vi "GetImageData.vi"(8 "error in (no error)":errorcluster, 11 "Image":T2) -> (0 "error out":errorcluster, 2 "ImageData Out":T1, 3 "Image out":T2)   [LabVIEW 2020]
uses:
  <vilib>/vision/Image Controls.llb/IMAQ Image.ctl
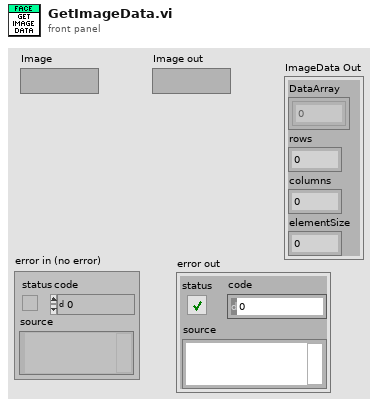
[diagram p1: front panel]
types:
  T1 = cluster{"DataArray":u8[], "rows":i32, "columns":i32, "elementSize":i32}
  T2 = typedef "IMAQ Image.ctl" = refnum<image>
  T3 = typedef "Image Type" = u32
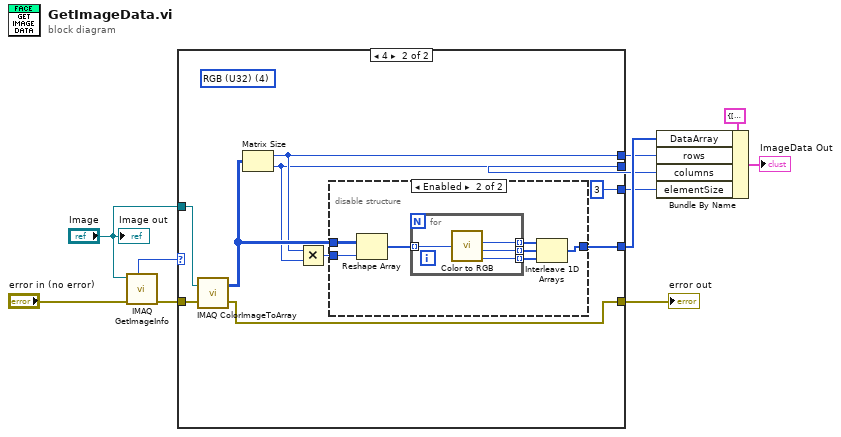
[diagram p0: block diagram]
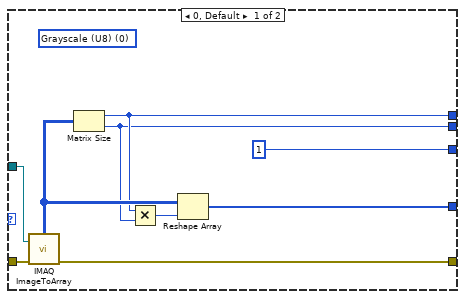
[diagram p2: hidden frame]
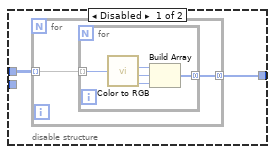
[diagram p3: hidden frame]
diagram:
  n1 = call "IMAQ GetImageInfo"("error in (no error)"="error in (no error)", "Image"="Image") -> ("error out"=w9:errorcluster, "Image Type"=w11:T3)  [unwired: 2 in, 6 out]
  n2 = case shown="4" w11 {
    tunnel: "Image" -> [w20 w29]
    tunnel: [w12 w28] -> w5
    tunnel: [1 3] -> w2
    tunnel: w9 -> [w18 w26]
    tunnel: [w17 w25] -> w7
    tunnel: [w14 w23] -> w4
    tunnel: [w13 w22] -> w3
    frame 0, Default {
      (unwired) T3 0 items=["Grayscale (U8)", "Grayscale (I16)", "Grayscale (SGL)", "Complex (CSG)", "RGB (U32)", "HSL (U32)", "RGB (U64)", "Grayscale (U16)"] ("Image Type")
      n3 = call "IMAQ ImageToArray"("error in (no error)"=w18, "Image"=w20) -> ("error out"=w17:errorcluster, "Image Pixels (U8)"=w16:u8[][])  [unwired: 2 in, 3 out]
      n4 = Matrix Size(0:w16) -> (1:w14:i32, 2:w13:i32)
      n5 = Multiply(x=w14, y=w13) -> (x*y=w15:i32)
      n6 = Reshape Array(w16, w15) -> (w12:u8[])
    }
    frame 4 {
      (unwired) T3 4 items=["Grayscale (U8)", "Grayscale (I16)", "Grayscale (SGL)", "Complex (CSG)", "RGB (U32)", "HSL (U32)", "RGB (U64)", "Grayscale (U16)"] ("Image Type")
      n7 = call "IMAQ ColorImageToArray"("Image"=w29, "error in (no error)"=w26) -> ("Image Pixels (U32)"=w24:u32[][], "error out"=w25:errorcluster)  [unwired: 2 in, 1 out]
      n8 = Matrix Size(0:w24) -> (1:w23:i32, 2:w22:i32)
      n9 = Multiply(x=w23, y=w22) -> (x*y=w21:i32)
      n10 = disable-structure shown="Enabled" {
        disable-tunnel: [w31 w39] -> w28
        disable-tunnel: w24 -> [w30 w45]
        disable-tunnel: w21 -> [_ w44]
        frame Disabled {
          n11 = for {
            tunnel: [w33] -> w31 mode=concatenating
            tunnel: w30 -> [w32] mode=indexing
            n12 = for {
              tunnel: w32 -> [w38] mode=indexing
              tunnel: [w34] -> w33 mode=concatenating
              n13 = call <vilib>:"Color to RGB.vi"("Color"=w38) -> ("R"=w37:u8, "G"=w36:u8, "B"=w35:u8)  [unwired: 1 out]
              n14 = Build Array(w37, w36, w35) -> (w34:u8[])
            }
          }
        }
        frame Enabled {
          n15 = Reshape Array(w45, w44) -> (w43:u32[])
          n16 = for {
            tunnel: w43 -> [w49] mode=indexing
            tunnel: [w48] -> w42 mode=indexing
            tunnel: [w47] -> w41 mode=indexing
            tunnel: [w46] -> w40 mode=indexing
            n17 = call <vilib>:"Color to RGB.vi"("Color"=w49) -> ("R"=w48:u8, "G"=w47:u8, "B"=w46:u8)  [unwired: 1 out]
          }
          n18 = Interleave 1D Arrays(w42, w41, w40) -> (w39:u8[])
        }
      }
    }
  }
  "error out" <- w7
  n19 = Bundle By Name(cluster=T1 {"DataArray"=[], "rows"=0, "columns"=0, "elementSize"=0} ("ImageData"), "DataArray"=w5, "rows"=w4, "columns"=w3, "elementSize"=w2) -> (→"ImageData Out":T1)
  "Image out" <- "Image"
